vi "Get String Value from HashTable.vi"(8 "error in (no error)":errorcluster caption="错误输入（无错误）", 10 "Name":string, 11 "Contstant Base 输入":refnum<class "Tag Data.lvclass"> caption="DNL_LabVIEW Object in") -> (0 "error out":errorcluster caption="错误输出", 2 "Value":string, 3 "Contstant Base 输出":refnum<class "Tag Data.lvclass"> caption="DNL_LabVIEW Object out")   [LabVIEW 2013, in "Tag Data.lvclass"]
uses:
  Tag Data.lvclass
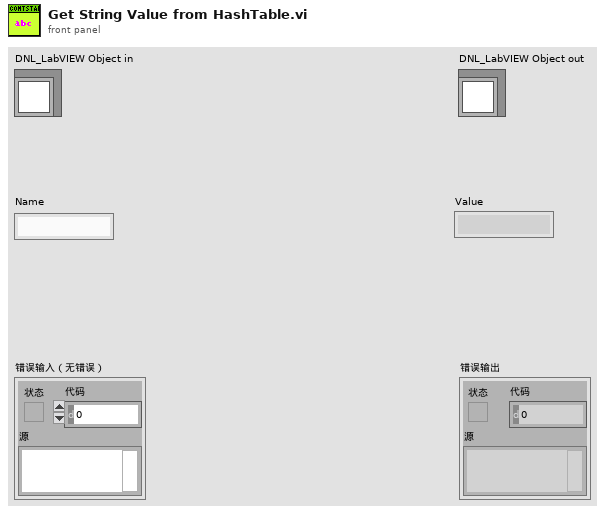
[diagram p1: front panel]
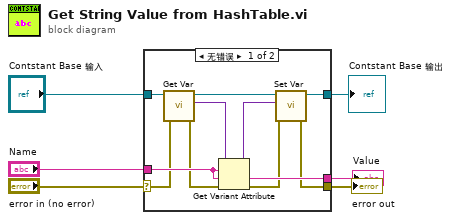
[diagram p0: block diagram]
diagram:
  n1 = case shown="无错误" "error in (no error)" {
    selector: "error in (no error)" -> [w10 w19]
    tunnel: [w7 w19] -> w5
    tunnel: [w11 w18] -> w3
    tunnel: "Contstant Base 输入" -> [w16 w18]
    tunnel: "Name" -> [w17 _]
    tunnel: [w12 _] -> w1
    frame No Error {
      n2 = call-dynamic "Get Var.vi"("error in (no error)"=w10, "Contstant Base输入"=w16) -> ("error out"=w9:errorcluster, "Var"=w14:variant, "Contstant Base输出"=w15:refnum<class "Tag Data.lvclass">)  [unwired: 7 in]
      n3 = Get Variant Attribute(Variant=w14, name=w17, default value (empty Variant)=w17, error in=w9) -> (duplicate Variant=w13:variant, value=w12:string, error out=w8:errorcluster)  [unwired: 1 out]
      n4 = call-dynamic "Set Var.vi"("error in (no error)"=w8, "Var"=w13, "Contstant Base输入"=w15) -> ("error out"=w7:errorcluster, "Contstant Base输出"=w11:refnum<class "Tag Data.lvclass">)  [unwired: 7 in]
    }
    frame Error {
    }
  }
  "error out" <- w5
  "Contstant Base 输出" <- w3
  "Value" <- w1
